vi "Read decryption.vi"(11 "Node in":refnum<class "Node.lvclass">) -> (2 "decryption":i64, 3 "Node out":refnum<class "Node.lvclass">)   [LabVIEW 2021, in "d20.lvlib" / "Node.lvclass"]
uses:
  Node.lvclass
  Node.lvclass/Node.ctl
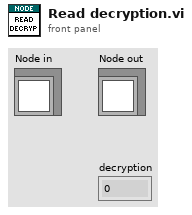
[diagram p1: front panel]
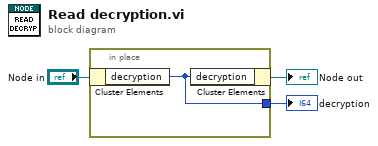
[diagram p0: block diagram]
diagram:
  n1 = in-place {
    in-place-border: [w4] -> w2
    n2 = in-place-cluster #1("Node in") -> ("decryption"=w4:i64)
    n3 = in-place-cluster #1("decryption"=w4) -> (→"Node out":refnum<class "Node.lvclass">)
  }
  "decryption" <- w2
